vi "DP-Isoresponse Contours.vi"(0 "Data matrix":dbl[][](array[numeric]), 1 "Which DP":enum16{"2f1-f2", "f2-f1"}(ring), 7 "F2 array":dbl[](array[numeric]), 11 "error in":errorcluster, 12 "criteria (dB)":dbl[](array[numeric])) -> (4 "DPGram":dbl[][](array[numeric]), 8 "F2 out":dbl[](array[numeric]), 10 "Noise floor data":dbl[][](array[numeric]), 13 "Array":T1(array[cluster]), 14 "IO Functions":T1(array[cluster]), 15 "error out":errorcluster)   [LabVIEW 2020]
uses:
  <vilib>/Analysis/NI_AALBase.lvlib
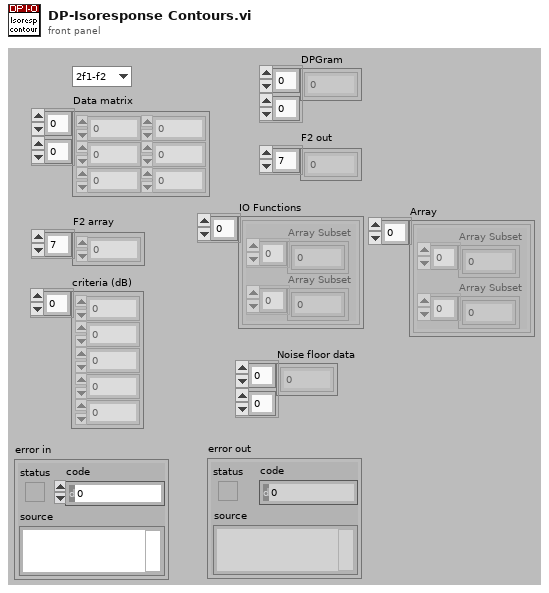
[diagram p1: front panel]
types:
  T1 = cluster{"Array Subset":dbl[], "Array Subset":dbl[]}[]
  T2 = cluster{"Array Subset":dbl[], "Array Subset":dbl[]}
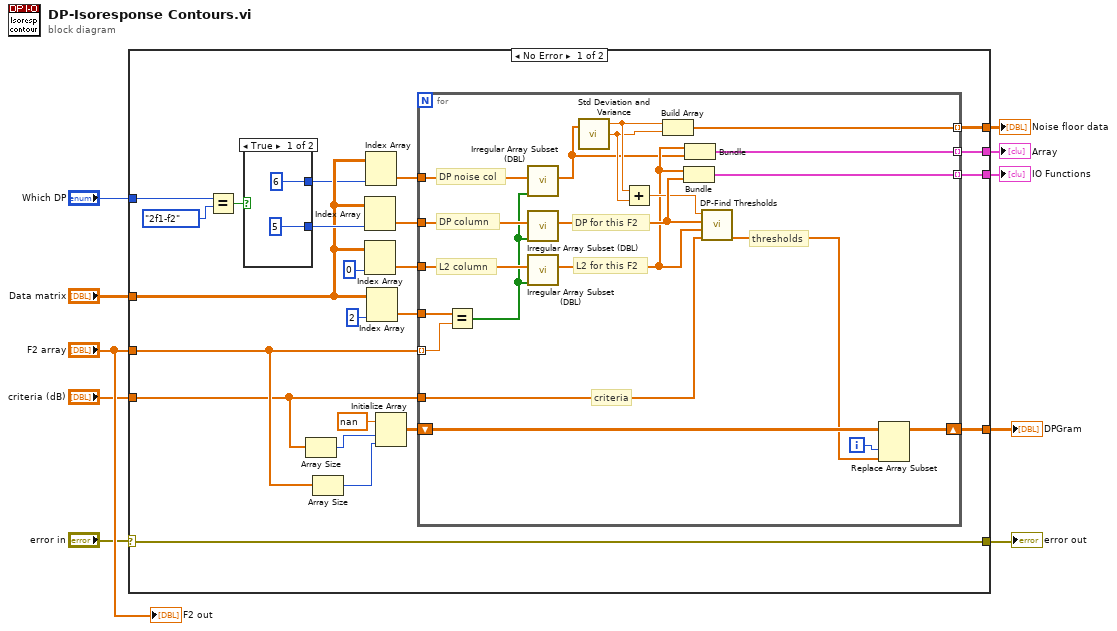
[diagram p0: block diagram]
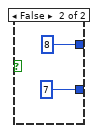
[diagram p2: hidden frame]
diagram:
  n1 = case shown="No Error" "error in" {
    selector: "error in" -> [w19 w58]
    tunnel: "F2 array" -> [w30 _]
    tunnel: "Data matrix" -> [w15 _]
    tunnel: [w23 _] -> w8
    tunnel: "criteria (dB)" -> [w22 _]
    tunnel: "Which DP" -> [w21 _]
    tunnel: [w19 w58] -> w4
    tunnel: [w18 _] -> w3
    tunnel: [w12 _] -> w2
    tunnel: [w11 _] -> w1
    frame No Error {
      n2 = Equal?(x=w21, y=enum16{"2f1-f2", "f2-f1"}."2f1-f2") -> (x = y?=w17:bool)
      n3 = case shown="True" w17 {
        tunnel: [5 ("disabled index (col)") 7 ("disabled index (col)")] -> w16
        tunnel: [6 ("disabled index (col)") 8 ("disabled index (col)")] -> w14
        frame True {
        }
        frame False {
        }
      }
      n4 = Array Size(array=w22) -> (size(s)=w31:i32)
      n5 = Array Size(array=w30) -> (size(s)=w32:i32)
      n6 = Index Array(array=w15, index (col)=w16) -> (element=w25:dbl[])  [unwired: 1 in]
      n7 = Index Array(array=w15, index (col)=0 ("index (row)")) -> (element=w27:dbl[])  [unwired: 1 in]
      n8 = Index Array(array=w15, index (col)=w14) -> (element=w13:dbl[])  [unwired: 1 in]
      n9 = Index Array(array=w15, index (col)=2 ("disabled index (col)")) -> (element=w28:dbl[])  [unwired: 1 in]
      n10 = Initialize Array(nan ("element"), w31, w32) -> (w24:dbl[][])
      n11 = for {
        tunnel: w30 -> [w57] mode=indexing
        tunnel: w28 -> [w56]
        tunnel: w27 -> [w55]
        tunnel: w25 -> [w54]
        tunnel: w22 -> [w44]
        shift-right: [w52] -> w23
        shift-left: w24 -> [w53]
        tunnel: [w51] -> w18 mode=indexing
        tunnel: w13 -> [w50]
        tunnel: [w48] -> w12 mode=indexing
        tunnel: [w40] -> w11 mode=indexing
        i -> [w39]
        # "DP noise col"
        # "thresholds"
        # "criteria"
        # "DP for this F2"
        # "L2 for this F2"
        # "DP column"
        # "L2 column"
        n12 = Equal?(x=w56, y=w57) -> (x = y?=w49:bool[])
        n13 = call "Irregular Array Subset (DBL).vi"("Mask"=w49, "Array"=w50) -> ("Array Subset"=w41:dbl[])  [unwired: 8 in, 1 out]
        n14 = call "Irregular Array Subset (DBL).vi"("Mask"=w49, "Array"=w54) -> ("Array Subset"=w45:dbl[])  [unwired: 8 in, 1 out]
        n15 = call "Irregular Array Subset (DBL).vi"("Mask"=w49, "Array"=w55) -> ("Array Subset"=w42:dbl[])  [unwired: 8 in, 1 out]
        n16 = call <vilib>:"Std Deviation and Variance.vi"("X"=w41) -> ("mean"=w47:dbl, "standard deviation"=w46:dbl)  [unwired: 1 in, 1 out]
        n17 = Add(x=w47, y=w46) -> (x+y=w43:dbl)
        n18 = Build Array(w47, w46) -> (w48:dbl[])
        n19 = Bundle("Array Subset"=w42, "Array Subset"=w45) -> (w51:T2)  [unwired: 1 in]
        n20 = Bundle("Array Subset"=w42, "Array Subset"=w41) -> (w40:T2)  [unwired: 1 in]
        n21 = call "DP-Find Thresholds.vi"("Criteria"=w44, "L2"=w42, "DP"=w45, "Noise criterion"=w43) -> ("Thresholds"=w38:dbl[])  [unwired: 7 in]
        n22 = Replace Array Subset(array=w53, new element=w38, index (col)=w39) -> (w52:dbl[][])  [unwired: 1 in]
      }
    }
    frame Error {
    }
  }
  "error out" <- w4
  "DPGram" <- w8
  "IO Functions" <- w3
  "Noise floor data" <- w2
  "Array" <- w1
  "F2 out" <- "F2 array"
